vi "From Boolean.vi"(0 "Value":bool, 1 "Key":string) -> (2 "Pair":refnum<class "Pair.lvclass">)   [LabVIEW 2018, in "Toolkit.lvlib" / "Data.lvlib" / "Pair.lvclass"]
uses:
  Pair.lvclass
  Pair.lvclass/Pair.ctl
  Boolean/Boolean.lvclass
  D:/Users/cfield/Code/Field R&D Services/Labstache/src/Toolkit/Data/Datum/Datum.lvclass
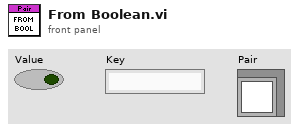
[diagram p1: front panel]
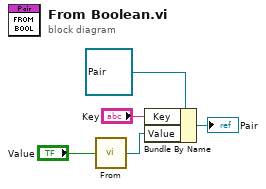
[diagram p0: block diagram]
diagram:
  n1 = call "From.vi"("Value"="Value") -> ("Boolean"=w2:refnum<class "Boolean.lvclass">)
  n2 = Bundle By Name(cluster=refnum<class "Pair.lvclass"> refnum ("Toolkit.lvlib:Data.lvlib:Pair.lvclass"), "Key"="Key", "Value"=w2) -> (→"Pair":refnum<class "Pair.lvclass">)
